vi "SMTP Email Keyed Array Clear.vi"(7 "array in":T1) -> (3 "array out":T1)   [LabVIEW 2012, in "NewNI_SMTPEmail.lvlib"]
uses:
  NewNI_SMTPEmail.lvlib
  SMTP Email Keyed Array.ctl
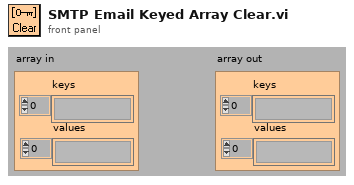
[diagram p1: front panel]
types:
  T1 = typedef "NewNI_SMTPEmail.lvlib/SMTP Email Keyed Array.ctl" = cluster{"keys":string[], "values":string[]}
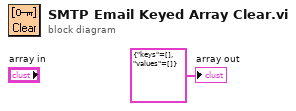
[diagram p0: block diagram]
diagram:
  "array out" <- cluster{"keys":string[], "values":string[]} {"keys"=[], "values"=[]} ("array out")
